vi "Swerve Sim.vi"() -> ()   [LabVIEW 2018]
panel:
  in  "stop":bool
  in  "Joystick R":dbl(slide) scale=-1.0..1.0
  in  "Joystick Y":dbl(slide) scale=-1.0..1.0
  in  "Joystick X":dbl(slide) scale=-1.0..1.0
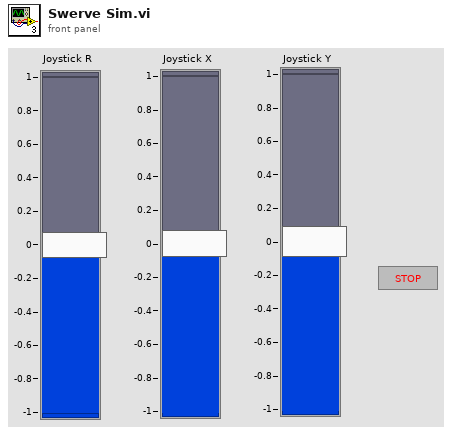
[diagram p1: front panel]
types:
  T1 = typedef "Robot Motion Commands.ctl" = cluster{"Front Right":T2, "Front Left":T2, "Rear Left":T2, "Rear Right":T2, "Drive Mode":T3}
  T2 = typedef "Motor Commands.ctl" = cluster{"Drive Power":dbl, "Drive Distance (in)":dbl, "Steer Power":dbl, "Steer Angle (deg)":dbl, "Steer Angle Error (deg)":dbl}
  T3 = typedef "Robot Drive Mode.ctl" = enum16{"Velocity", "Distance"}
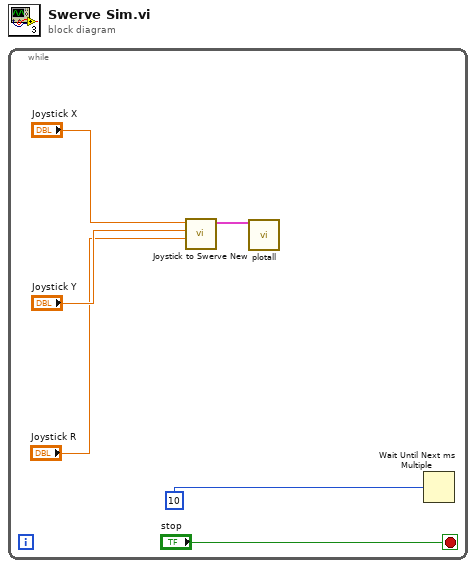
[diagram p0: block diagram]
diagram:
  n1 = while {
    stop <- "stop" stop-if-true
    n2 = call "Joystick to Swerve New.vi"("Joystick R"="Joystick R", "Joystick Y"="Joystick Y", "Joystick X"="Joystick X") -> ("Robot Motion Commands"=w1:T1)  [unwired: 8 in]
    n3 = call "plotall.vi"("Robot Motion Commands"=w1) -> ()  [unwired: 11 in]
    n4 = Wait Until Next ms Multiple(millisecond multiple=u32 10 ("millisecond timer value")) -> ()  [unwired: 1 out]
  }
